vi "UnderlineDecorator_Create.vi"(8 "Error In":errorcluster, 11 "reference in":refnum<class "UnderlineDecorator.lvclass">) -> (0 "Error Out":errorcluster, 3 "reference out":refnum<class "UnderlineDecorator.lvclass">)   [LabVIEW 2024, in "UnderlineDecorator.lvclass"]
uses:
  UnderlineDecorator.lvclass/UnderlineDecorator.ctl
  UnderlineDecorator.lvclass
  TextDecorator/TextDecorator.lvclass
  C:/Users/burakkorkmaz/Desktop/Leveling/labview-design-patterns/Decorator Pattern/Labview/TextDecorator/TextDecorator.lvclass
  C:/Users/burakkorkmaz/Desktop/Leveling/labview-design-patterns/Decorator Pattern/Labview/IText/IText.lvclass
  C:/Users/burakkorkmaz/Desktop/Leveling/labview-design-patterns/Decorator Pattern/Labview/UnderlineDecorator/UnderlineDecorator.lvclass
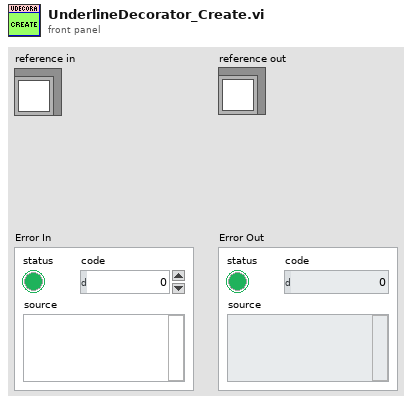
[diagram p1: front panel]
types:
  T1 = typedef "UnderlineDecorator.lvclass/ObjectAttributes.ctl" = cluster{"None":bool}
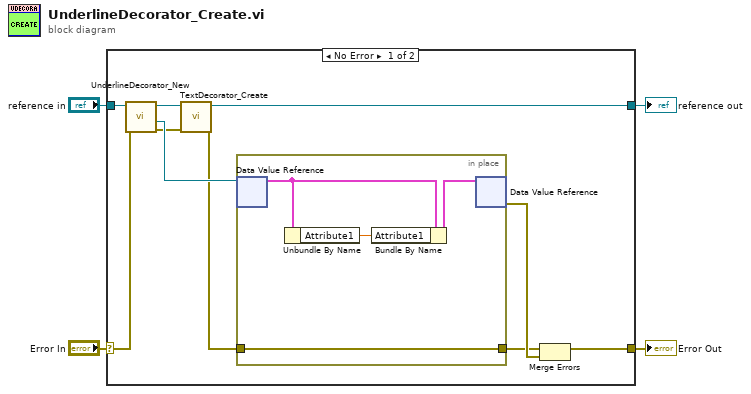
[diagram p0: block diagram]
diagram:
  n1 = case shown="No Error" "Error In" {
    selector: "Error In" -> [w10 w20]
    tunnel: [w8 w20] -> w3
    tunnel: "reference in" -> [w12 w19]
    tunnel: [w7 w19] -> w1
    frame No Error {
      n2 = call "UnderlineDecorator_New.vi"("Error In"=w10, "reference in"=w12) -> ("Error Out"=w11:errorcluster, "DVRRefOut"=w14:refnum<data-value>, "reference out"=w13:refnum<class "UnderlineDecorator.lvclass">)  [unwired: 6 in, 1 out]
      n3 = call "TextDecorator_Create.vi"("Error In"=w11, "reference in"=w13) -> ("Error Out"=w6:errorcluster, "reference out"=w7:refnum<class "UnderlineDecorator.lvclass">)  [unwired: 8 in]
      n4 = in-place {
        in-place-border: w6 -> [w15]
        in-place-border: [w15] -> w5
        n5 = in-place-dvr #1(w14) -> (w17:T1)  [unwired: 1 out]
        n6 = Unbundle By Name(w17) -> ("Attribute1"=w16:dbl)
        n7 = Bundle By Name(cluster=w17, "Attribute1"=w16) -> (w18:T1)
        n8 = in-place-dvr #1(w18) -> (w9:errorcluster)  [unwired: 1 out]
      }
      n9 = Merge Errors(w5, w9) -> (w8:errorcluster)
    }
    frame Error {
    }
  }
  "Error Out" <- w3
  "reference out" <- w1
